vi "Handle1.vi"(8 "error in (no error)":errorcluster, 11 "Sync Box in":refnum<class "Sync Box.lvclass">) -> (0 "error out":errorcluster, 3 "Sync Box out":refnum<class "Sync Box.lvclass">)   [LabVIEW 2018]
uses:
  Comm/Stream/Stream.lvclass
  Sync Box.lvclass
  C:/Users/observer/Desktop/Sparc4GUI - 21-01-2021/SPARC4_GUI/Server/Server.lvclass
  Device/Device.lvclass
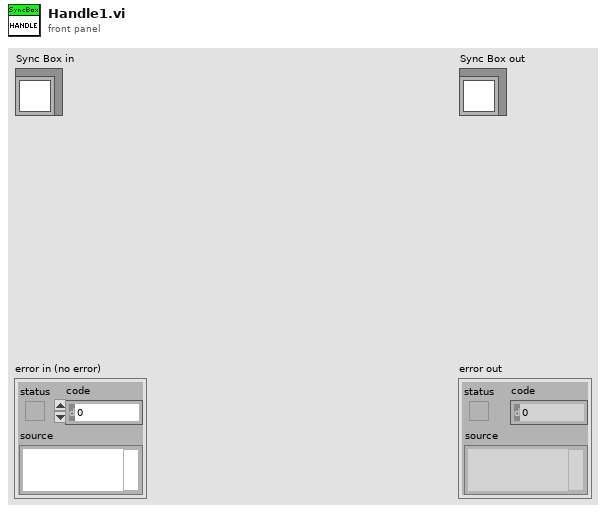
[diagram p1: front panel]
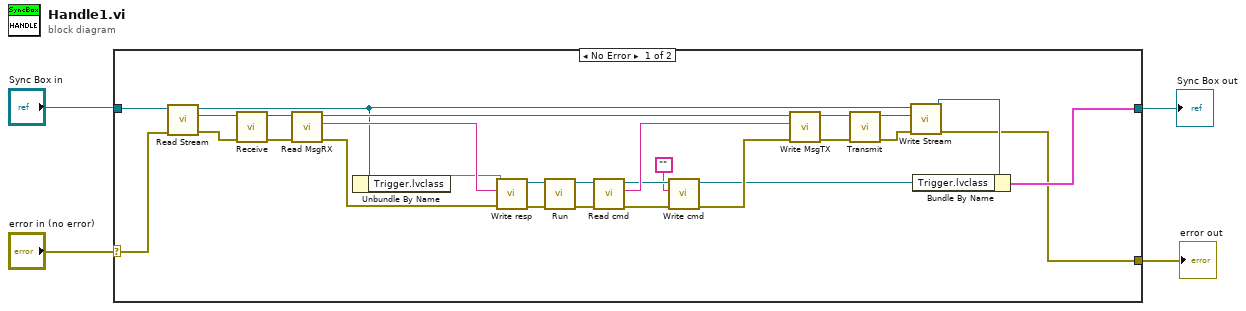
[diagram p0: block diagram]
diagram:
  n1 = case shown="No Error" "error in (no error)" {
    selector: "error in (no error)" -> [w30 w34]
    tunnel: [w15 w34] -> w1
    tunnel: [w29 w33] -> w2
    tunnel: "Sync Box in" -> [w14 w33]
    frame No Error {
      n2 = call-dynamic "Read Stream.vi"("error in (no error)"=w30, "Server in"=w14) -> ("error out"=w31:errorcluster, "Stream.lvclass"=w32:refnum<class "Stream.lvclass">, "Server out"=w19:refnum<class "Sync Box.lvclass">)  [unwired: 7 in]
      n3 = call-dynamic "Receive.vi"("error in (no error)"=w31, "Stream in"=w32) -> ("error out"=w28:errorcluster, "Stream out"=w27:refnum<class "Stream.lvclass">)  [unwired: 8 in]
      n4 = call-dynamic "Read MsgRX.vi"("error in (no error)"=w28, "Comm in"=w27) -> ("error out"=w25:errorcluster, "MsgRX"=w26:string, "Comm out"=w24:refnum<class "Stream.lvclass">)  [unwired: 7 in]
      n5 = Unbundle By Name(w19) -> ("Trigger.lvclass"=w6)
      n6 = call-dynamic "Write resp.vi"("error in (no error)"=w25, "resp"=w26, "Device in"=w6) -> ("error out"=w13:errorcluster, "Device out"=w12:refnum<class "Device.lvclass">)  [unwired: 7 in]
      n7 = call-dynamic "Run.vi"("error in (no error)"=w13, "Device in"=w12) -> ("error out"=w10:errorcluster, "Device out"=w11:refnum<class "Device.lvclass">)  [unwired: 8 in]
      n8 = call-dynamic "Read cmd.vi"("error in (no error)"=w10, "Device in"=w11) -> ("error out"=w8:errorcluster, "cmd"=w23:string, "Device out"=w9:refnum<class "Device.lvclass">)  [unwired: 7 in]
      n9 = call-dynamic "Write cmd.vi"("error in (no error)"=w8, "cmd"="", "Device in"=w9) -> ("error out"=w22:errorcluster, "Device out"=w5:refnum<class "Device.lvclass">)  [unwired: 7 in]
      n10 = call-dynamic "Write MsgTX.vi"("error in (no error)"=w22, "MsgTX"=w23, "Comm in"=w24) -> ("error out"=w20:errorcluster, "Comm out"=w21:refnum<class "Stream.lvclass">)  [unwired: 7 in]
      n11 = call-dynamic "Transmit.vi"("error in (no error)"=w20, "Stream in"=w21) -> ("error out"=w16:errorcluster, "Stream out"=w18:refnum<class "Stream.lvclass">)  [unwired: 8 in]
      n12 = call-dynamic "Write Stream.vi"("error in (no error)"=w16, "Stream.lvclass"=w18, "Server in"=w19) -> ("error out"=w15:errorcluster, "Server out"=w17:refnum<class "Sync Box.lvclass">)  [unwired: 7 in]
      n13 = Bundle By Name(cluster=w17, "Trigger.lvclass"=w5) -> (w29:cluster{})
    }
    frame Error {
    }
  }
  "error out" <- w1
  "Sync Box out" <- w2
